vi "Load Plot Group Prefs.vi"(10 "Hierarchy":string[](array[string]), 11 "Pref Group in":refnum<class "Pref Group.lvclass">) -> (2 "Plot Group Config":T1)   [LabVIEW 2020, in "VolatusGUI.lvlib" / "Historian Charting Manager.lvclass"]
uses:
  Historian Charting Manager.lvclass
  Historian Charting Manager.lvclass/Historian Charting Manager.ctl
  lv-userprefs/User Prefs/Pref Group/Pref Group.lvclass
  X-Axis Type.ctl
  Scale.ctl
  Plot Config.ctl
  Plot Group Config.ctl
  VolatusGUIElements/VolatusGUIElements.lvlib
  lv-vecto/Vecto/Vecto.lvlib
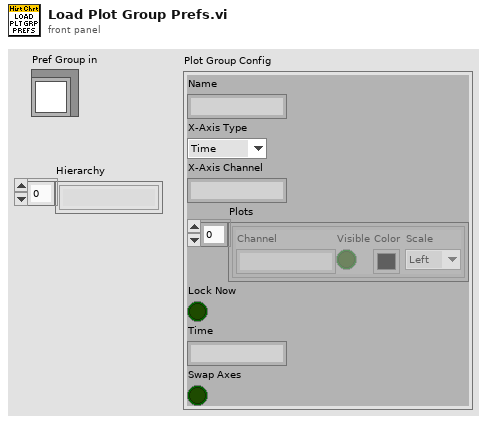
[diagram p1: front panel]
types:
  T1 = typedef "VolatusGUI.lvlib/Historian Charting Manager.lvclass/Plot Group Config.ctl" = cluster{"Name":string, "X-Axis Type":T2, "X-Axis Channel":string, "Plots":T3[], "Lock Now":bool, "Time":string, "Swap Axes":bool}
  T2 = typedef "VolatusGUI.lvlib/Historian Charting Manager.lvclass/X-Axis Type.ctl" = enum16{"Time", "Channel"}
  T3 = typedef "VolatusGUI.lvlib/Historian Charting Manager.lvclass/Plot Config.ctl" = cluster{"Channel":string, "Visible":bool, "Color":u32, "Scale":T4}
  T4 = typedef "VolatusGUI.lvlib/Historian Charting Manager.lvclass/Scale.ctl" = enum16{"Left", "Right"}
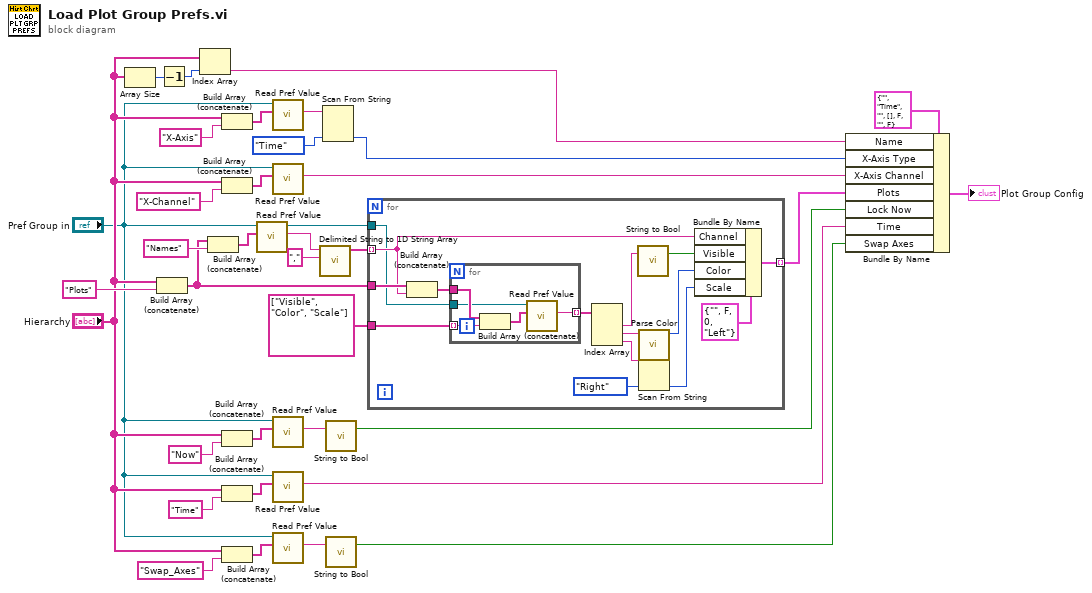
[diagram p0: block diagram]
diagram:
  n1 = Array Size(array="Hierarchy") -> (size(s)=w26:i32)
  n2 = Build Array (concatenate)("Hierarchy", "Plots") -> (w29:string[])
  n3 = Decrement(x=w26) -> (x-1=w25:i32)
  n4 = Index Array(array="Hierarchy", index=w25) -> (element=w24:string)
  n5 = Build Array (concatenate)(w29, "Names") -> (w34:string[])
  n6 = Build Array (concatenate)("Hierarchy", "X-Axis") -> (w20:string[])
  n7 = Build Array (concatenate)("Hierarchy", "X-Channel") -> (w16:string[])
  n8 = Build Array (concatenate)("Hierarchy", "Now") -> (w12:string[])
  n9 = Build Array (concatenate)("Hierarchy", "Time") -> (w9:string[])
  n10 = Build Array (concatenate)("Hierarchy", "Swap_Axes") -> (w5:string[])
  n11 = call "Read Pref Value.vi"("Pref Hierarchy"=w34, "Pref Group in"="Pref Group in") -> ("Value"=w33:string, "Pref Group out"=w31:refnum<class "Pref Group.lvclass">)  [unwired: 7 in, 1 out]
  n12 = call "Read Pref Value.vi"("Pref Hierarchy"=w20, "Pref Group in"="Pref Group in") -> ("Value"=w19:string)  [unwired: 7 in, 2 out]
  n13 = call "Read Pref Value.vi"("Pref Hierarchy"=w16, "Pref Group in"="Pref Group in") -> ("Value"=w14:string)  [unwired: 7 in, 2 out]
  n14 = call "Read Pref Value.vi"("Pref Hierarchy"=w12, "Pref Group in"="Pref Group in") -> ("Value"=w11:string)  [unwired: 7 in, 2 out]
  n15 = call "Read Pref Value.vi"("Pref Hierarchy"=w9, "Pref Group in"="Pref Group in") -> ("Value"=w7:string)  [unwired: 7 in, 2 out]
  n16 = call "Read Pref Value.vi"("Pref Hierarchy"=w5, "Pref Group in"="Pref Group in") -> ("Value"=w2:string)  [unwired: 7 in, 2 out]
  n17 = call <vilib>:"Delimited String to 1D String Array.vi"("delimiter"=",", "delimited string"=w33) -> ("string array"=w30:string[])  [unwired: 9 in]
  n18 = Scan From String(input string=w19, default 1=X-Axis_Type."Time" ("X-Axis Type")) -> (output 1=w17:T2)  [unwired: 3 in, 3 out]
  n19 = call "String to Bool.vi"("String"=w11) -> ("Bool"=w10:bool)  [unwired: 2 in]
  n20 = call "String to Bool.vi"("String"=w2) -> ("Bool"=w1:bool)  [unwired: 2 in]
  n21 = for {
    tunnel: w31 -> [w47]
    tunnel: w30 -> [w49] mode=indexing
    tunnel: w29 -> [w51]
    tunnel: string[] ["Visible", "Color", "Scale"] -> [w46]
    tunnel: [w37] -> w22 mode=indexing
    n22 = Build Array (concatenate)(w51, w49) -> (w48:string[])
    n23 = for {
      tunnel: w48 -> [w55]
      tunnel: w47 -> [w54]
      tunnel: w46 -> [w56] mode=indexing
      tunnel: [w52] -> w45 mode=indexing
      n24 = Build Array (concatenate)(w55, w56) -> (w53:string[])
      n25 = call "Read Pref Value.vi"("Pref Hierarchy"=w53, "Pref Group in"=w54) -> ("Value"=w52:string)  [unwired: 7 in, 2 out]
    }
    n26 = Index Array(array=w45) -> (element #1=w39:string, element #2=w44:string, element #3=w42:string)  [unwired: 3 in]
    n27 = call "String to Bool.vi"("String"=w39) -> ("Bool"=w38:bool)  [unwired: 2 in]
    n28 = call "Parse Color.vi"("Color String"=w44) -> ("Color"=w43:u32)  [unwired: 9 in, 1 out]
    n29 = Scan From String(input string=w42, default 1=Scale."Right" ("Scale")) -> (output 1=w41:T4)  [unwired: 3 in, 3 out]
    n30 = Bundle By Name(cluster=T3 {"Channel"="", "Visible"=FALSE, "Color"=0, "Scale"=enum."Left"} ("Plot Config"), "Channel"=w49, "Visible"=w38, "Color"=w43, "Scale"=w41) -> (w37:T3)
  }
  n31 = Bundle By Name(cluster=T1 {"Name"="", "X-Axis Type"=enum."Time", "X-Axis Channel"="", "Plots"=[], "Lock Now"=FALSE, "Time"="", "Swap Axes"=FALSE} ("Plot Group Config"), "Name"=w24, "X-Axis Type"=w17, "X-Axis Channel"=w14, "Plots"=w22, "Lock Now"=w10, "Time"=w7, "Swap Axes"=w1) -> (→"Plot Group Config":T1)
